vi "Excel_Set_Header_Font.vi"(0 "left footer text in":string, 1 "font":T1 {"font size" format="%0.2f"; "strike through" items=["Strk Unchanged", "Strk Yes", "Strk No"]; "underline" items=["Und Unchanged", "Und Yes", "Und No"]; "italic" items=["Ital Unchanged", "Ital Yes", "Ital No"]; "bold" items=["Bold Unchanged", "Bold Yes", "Bold No"]}, 2 "center footer text in":string, 3 "right footer text in":string) -> (6 "left footer text out":string, 7 "center footer text out":string, 9 "right footer text out":string)   [LabVIEW 2017, in "NI_ReportGenerationToolkit.lvlib"]
uses:
  <vilib>/addons/_office/NI_ReportGenerationToolkit.lvlib
  <vilib>/addons/_office/_exclsub.llb/font.ctl
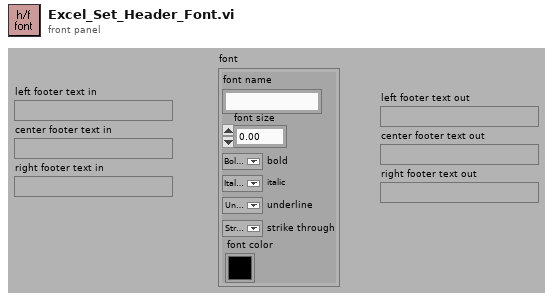
[diagram p1: front panel]
types:
  T1 = typedef "NI_ReportGenerationToolkit.lvlib/font.ctl" = cluster{"font name":string, "font size":dbl, "bold":u16, "italic":u16, "underline":u16, "strike through":u16, "font color":u32}
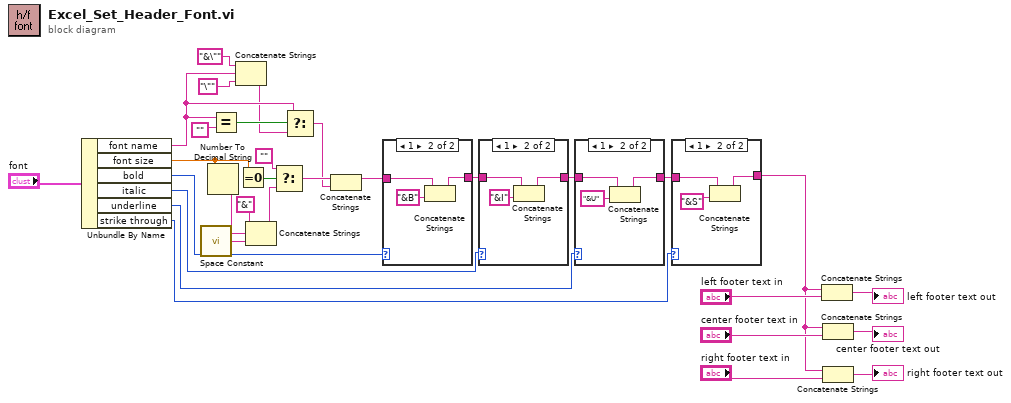
[diagram p0: block diagram]
diagram:
  n1 = Unbundle By Name("font") -> ("font name"=w8:string, "font size"=w15:dbl, "bold"=w29:u16, "italic"=w28:u16, "underline"=w27:u16, "strike through"=w26:u16)
  n2 = call <vilib>:"Space Constant.vi"() -> ("String"=w1:string)
  n3 = Number To Decimal String(number=w15) -> (decimal integer string=w5:string)  [unwired: 1 out]
  n4 = Equal?(x=w8, y="") -> (x = y?=w9:bool)
  n5 = Concatenate Strings("&\"" ("Substring"), w8, "\"" ("Substring")) -> (w7:string)
  n6 = Equal To 0?(x=w15) -> (x = 0?=w13:bool)
  n7 = Concatenate Strings("&" ("Substring"), w5, w1) -> (w3:string)
  n8 = Select(t="", s=w13, f=w3) -> (s? t:f=w11:string)
  n9 = Select(t=w8, s=w9, f=w7) -> (s? t:f=w6:string)
  n10 = Concatenate Strings(w11, w6) -> (w30:string)
  n11 = case shown="1" w29 {
    tunnel: w30 -> [w32 w35]
    tunnel: [w32 w33] -> w25
    frame 0, Default {
    }
    frame 1 {
      n12 = Concatenate Strings(w35, "&B" ("Substring")) -> (w33:string)
    }
  }
  n13 = case shown="1" w28 {
    tunnel: w25 -> [w36 w38]
    tunnel: [w36 w37] -> w24
    frame 0, Default {
    }
    frame 1 {
      n14 = Concatenate Strings(w38, "&I" ("Substring")) -> (w37:string)
    }
  }
  n15 = case shown="1" w27 {
    tunnel: w24 -> [w40 w42]
    tunnel: [w40 w41] -> w23
    frame 0, Default {
    }
    frame 1 {
      n16 = Concatenate Strings(w42, "&U" ("Substring")) -> (w41:string)
    }
  }
  n17 = case shown="1" w26 {
    tunnel: w23 -> [w44 w46]
    tunnel: [w44 w45] -> w16
    frame 0, Default {
    }
    frame 1 {
      n18 = Concatenate Strings(w46, "&S" ("Substring")) -> (w45:string)
    }
  }
  n19 = Concatenate Strings(w16, "left footer text in") -> (→"left footer text out":string)
  n20 = Concatenate Strings(w16, "center footer text in") -> (→"center footer text out":string)
  n21 = Concatenate Strings(w16, "right footer text in") -> (→"right footer text out":string)
